vi "Front IO Panel.vi"(11 "Full System Configuration":T1={"Rack"=enum."15U; 1-Phase; 16A; 100-240V", "Middle Rail"=enum."None", "Ballast"={"Main"=0, "Small"=0, "Side"=0}, "Front Panel I/O"={"EMO Button"=FALSE, "USB 3.0"=FALSE, "Display"=FALSE, "1st USB 2.0"=FALSE, "2nd USB 2.0"=FALSE, "Ethernet 3"=FALSE, "EMO Extension (3rd Party)"=FALSE, "EMO Extension (Rack In & Out)"=FALSE, "Aux Dual C13 QAC Outlets"=FALSE, "Residual-current Circuit Breaker"=FALSE, "Serial"=FALSE, "GPIB"=FALSE}, "Rear Panel I/O"={"Rear Panel I/O Configuration"=enum."Blank Panel", "EMO Button"=FALSE, "Power, Status & Banana Ground"=FALSE, "Ethernet 2"=FALSE, "Display"=FALSE, "USB 3.0"=FALSE, "DIO"=FALSE, "GPIB"=FALSE, "Aux Dual C13 QAC Outlets"=FALSE, "Residual-current Circuit Breaker"=FALSE, "Serial"=FALSE, "SMA"=FALSE}, "Miscellaneous Options"={"Eyebolts"=FALSE, "Tower Light"=FALSE, "Top/Side Monitor Mount Kit"=FALSE, "24\" Monitor"=FALSE, "Keyboard & Mouse"=FALSE, "Secondary Ethernet Switch"=FALSE, "Extra USB Hub"=FALSE, "USB-6509"=FALSE, "Front Door"=enum."38U (Solid) IG", "Primary Ethernet Switch"=enum."Item 0", "Use Posture"=enum."Item 0"}, "Accessories"={"Screw Type"=enum."10-32", "Cage Nuts & Screws"=0.0, "Filler Panel Color"=enum."Interface Gray", "1U"=0.0, "2U"=0.0, "3U"=0.0}} {"Ballast"."Side" max=5 step=1; "Ballast"."Small" max=5 step=1; "Ballast"."Main" max=5 step=1}) -> (3 "Array":T13[](array[typedef]))   [LabVIEW 2023]
uses:
  Option Type Defs/Parts List.ctl
  Option Type Defs/Full System Configuration.ctl
  Option Type Defs/Rack.ctl
  Option Type Defs/Middle Rail.ctl
  Option Type Defs/Ballast.ctl
  Option Type Defs/Front Panel IO.ctl
  Option Type Defs/Rear Panel IO.ctl
  Option Type Defs/Rear Panel IO Configuration.ctl
  Option Type Defs/Miscellaneous Options.ctl
  Option Type Defs/Front Door.ctl
  Option Type Defs/Accessories.ctl
  Option Type Defs/Screw Types.ctl
  Option Type Defs/Filler Panel Color.ctl
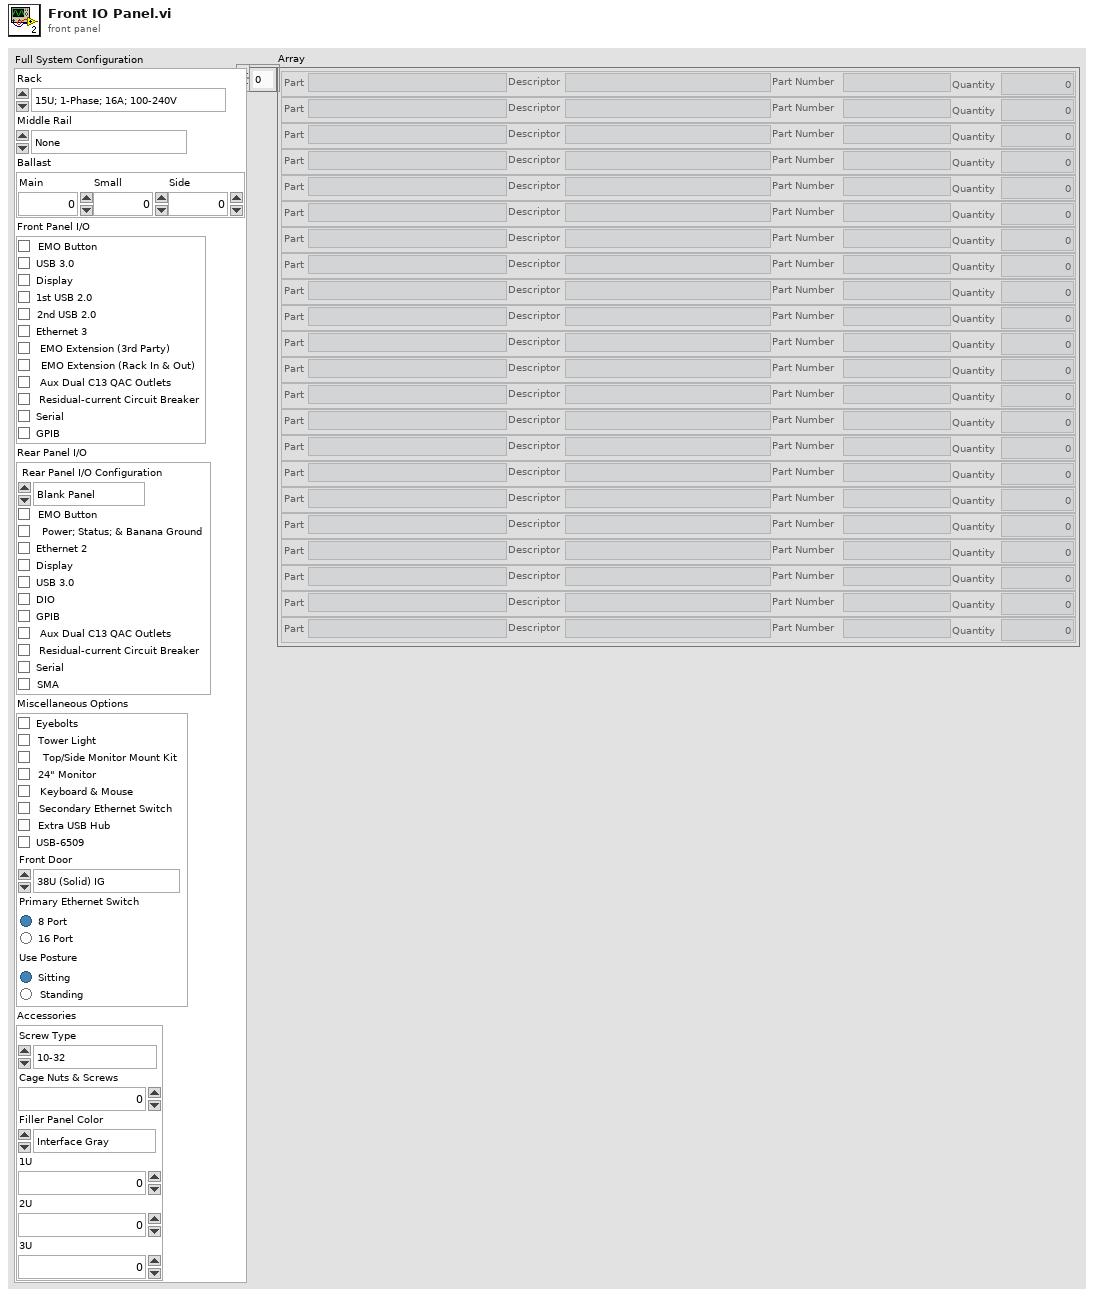
[diagram p1: front panel]
types:
  T1 = typedef "Full System Configuration.ctl" = cluster{"Rack":T2, "Middle Rail":T3, "Ballast":T4, "Front Panel I/O":T5, "Rear Panel I/O":T6, "Miscellaneous Options":T8, "Accessories":T10}
  T2 = typedef "Rack.ctl" = enum16{"15U; 1-Phase; 16A; 100-240V", "15U; 1-Phase; 24A; 100-240V", "38U; 3-Phase Delta; 50A; 200-240V", "38U; 1-Phase; 24A; 100-120V", "38U; 3-Phase Wye; 50A; 200-240V", "38U; 3-Phase Delta; 50A; 380-480V", "38U; 3-Phase Delta; 32A; 200-240V", "38U; 3-Phase Wye; 16A; 100-240V", "44U; 1-Phase; 24A; 100-240V", "44U; 3-Phase Delta; 32A; 200-240V"}
  T3 = typedef "Middle Rail.ctl" = enum16{"None", "Flip Side Rear; D=168.83mm", "Parallel Rear; D=145mm", "Flip Side Front; D=145mm", "Parallel Front; D=145mm"}
  T4 = typedef "Ballast.ctl" = cluster{"Main":u16, "Small":u16, "Side":u16}
  T5 = typedef "Front Panel IO.ctl" = cluster{"EMO Button":bool, "USB 3.0":bool, "Display":bool, "1st USB 2.0":bool, "2nd USB 2.0":bool, "Ethernet 3":bool, "EMO Extension (3rd Party)":bool, "EMO Extension (Rack In & Out)":bool, "Aux Dual C13 QAC Outlets":bool, "Residual-current Circuit Breaker":bool, "Serial":bool, "GPIB":bool}
  T6 = typedef "Rear Panel IO.ctl" = cluster{"Rear Panel I/O Configuration":T7, "EMO Button":bool, "Power, Status & Banana Ground":bool, "Ethernet 2":bool, "Display":bool, "USB 3.0":bool, "DIO":bool, "GPIB":bool, "Aux Dual C13 QAC Outlets":bool, "Residual-current Circuit Breaker":bool, "Serial":bool, "SMA":bool}
  T7 = typedef "Rear Panel IO Configuration.ctl" = enum16{"Blank Panel", "Fully Populated Panel", "Custom Panel"}
  T8 = typedef "Miscellaneous Options.ctl" = cluster{"Eyebolts":bool, "Tower Light":bool, "Top/Side Monitor Mount Kit":bool, "24\" Monitor":bool, "Keyboard & Mouse":bool, "Secondary Ethernet Switch":bool, "Extra USB Hub":bool, "USB-6509":bool, "Front Door":T9, "Primary Ethernet Switch":enum32{"Item 0", "Item 1"}, "Use Posture":enum32{"Item 0", "Item 1"}}
  T9 = typedef "Front Door.ctl" = enum16{"None", "38U (Solid) IG", "38U (Solid) EG", "38U: Top 14U (Solid) IG", "38U (Clear) IG", "44U (Solid) IG", "44U (Solid) EG"}
  T10 = typedef "Accessories.ctl" = cluster{"Screw Type":T11, "Cage Nuts & Screws":dbl, "Filler Panel Color":T12, "1U":dbl, "2U":dbl, "3U":dbl}
  T11 = typedef "Screw Types.ctl" = enum16{"None", "M6 (Most Common)", "10-32", "12-24"}
  T12 = typedef "Filler Panel Color.ctl" = enum16{"None", "Interface Gray", "Environmental Gray"}
  T13 = typedef "Parts List.ctl" = cluster{"Part":string, "Descriptor":string, "Part Number":string, "Quantity":dbl}
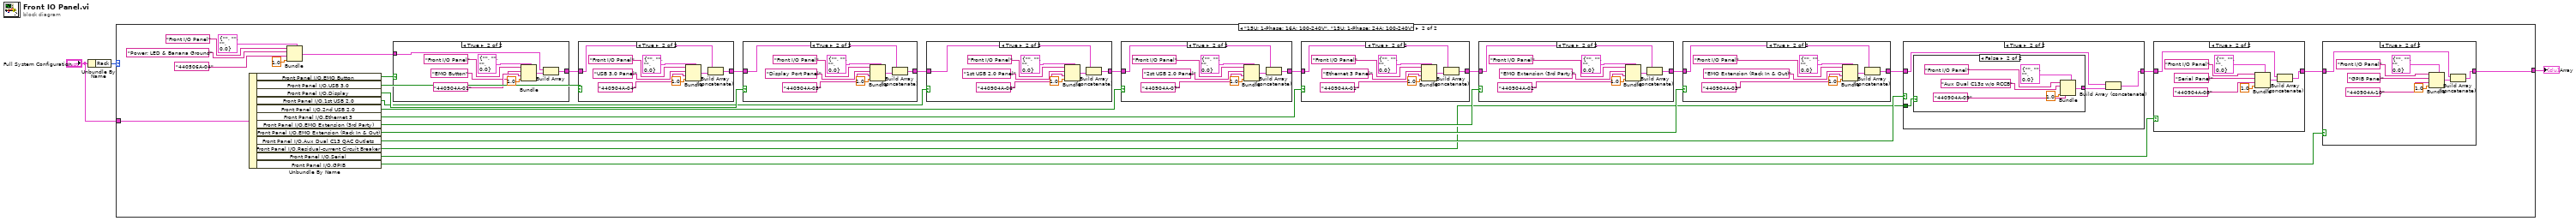
[diagram p0: block diagram]
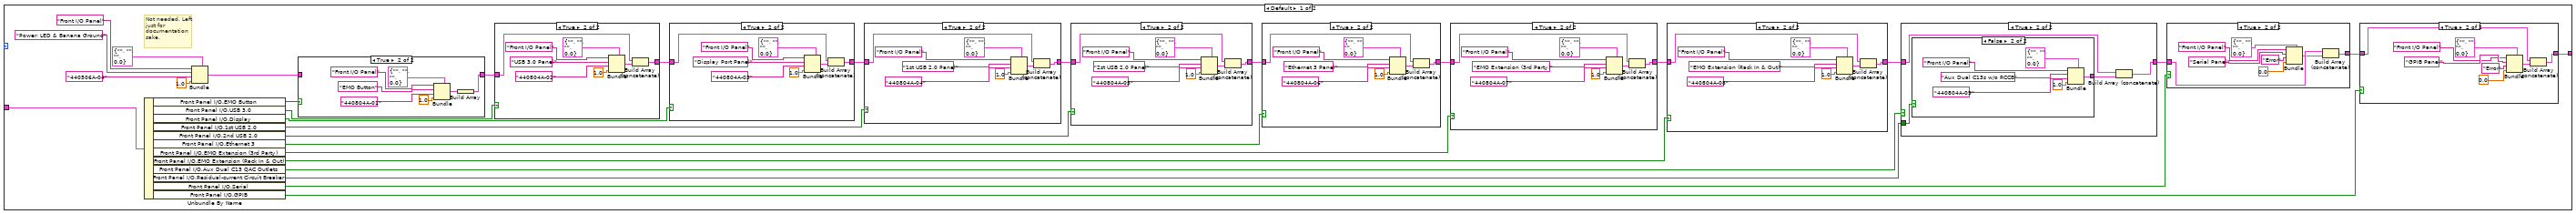
[diagram p2: hidden frame]
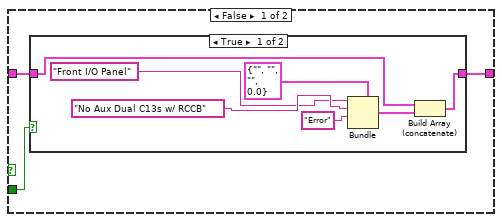
[diagram p5: hidden frame]
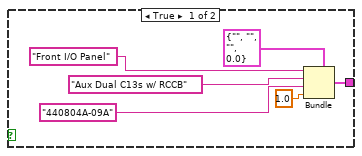
[diagram p7: hidden frame]
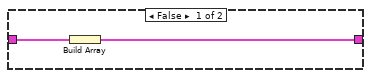
[diagram p15: hidden frame]
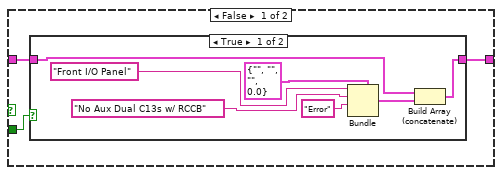
[diagram p18: hidden frame]
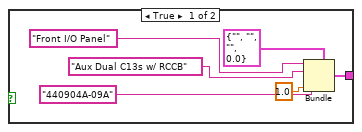
[diagram p20: hidden frame]
diagram:
  n1 = Unbundle By Name("Full System Configuration") -> ("Rack"=w3:T2)
  n2 = case shown="\"15U; 1-Phase; 16A; 100-240V\", \"15U; 1-Phase; 24A; 100-240V\"" w3 {
    tunnel: [w5 w152] -> w2
    tunnel: "Full System Configuration" -> [w28 w175]
    frame Default {
      # "Not needed. Left just for documentation sake."
      n3 = Unbundle By Name(w28) -> ("Front Panel I/O.EMO Button"=w27:bool, "Front Panel I/O.USB 3.0"=w26:bool, "Front Panel I/O.Display"=w23:bool, "Front Panel I/O.1st USB 2.0"=w21:bool, "Front Panel I/O.2nd USB 2.0"=w20:bool, "Front Panel I/O.Ethernet 3"=w18:bool, "Front Panel I/O.EMO Extension (3rd Party)"=w15:bool, "Front Panel I/O.EMO Extension (Rack In & Out)"=w13:bool, "Front Panel I/O.Aux Dual C13 QAC Outlets"=w12:bool, "Front Panel I/O.Residual-current Circuit Breaker"=w11:bool, "Front Panel I/O.Serial"=w7:bool, "Front Panel I/O.GPIB"=w6:bool)
      n4 = Bundle(cluster=T13 {"Part"="", "Descriptor"="", "Part Number"="", "Quantity"=0.0}, "Part"="Front I/O Panel", "Descriptor"="Power; LED & Banana Ground", "Part Number"="440506A-04", "Quantity"=1.0) -> (w33:T13)
      n5 = case shown="True" w27 {
        tunnel: w33 -> [w143 _]
        tunnel: [w142 w150] -> w25
        frame False {
          n6 = Build Array(w143) -> (w142:T13[])
        }
        frame True {
          n7 = Bundle(cluster=T13 {"Part"="", "Descriptor"="", "Part Number"="", "Quantity"=0.0}, "Part"="Front I/O Panel", "Descriptor"="EMO Button", "Part Number"="440804A-01", "Quantity"=1.0) -> (w145:T13)
          n8 = Build Array(w145) -> (w150:T13[])
        }
      }
      n9 = case shown="True" w26 {
        tunnel: w25 -> [w133 w141]
        tunnel: [w133 w140] -> w24
        frame False {
        }
        frame True {
          n10 = Bundle(cluster=T13 {"Part"="", "Descriptor"="", "Part Number"="", "Quantity"=0.0}, "Part"="Front I/O Panel", "Descriptor"="USB 3.0 Panel", "Part Number"="440804A-02", "Quantity"=1.0) -> (w135:T13)
          n11 = Build Array (concatenate)(w141, w135) -> (w140:T13[])
        }
      }
      n12 = case shown="True" w23 {
        tunnel: w24 -> [w124 w132]
        tunnel: [w124 w131] -> w22
        frame False {
        }
        frame True {
          n13 = Bundle(cluster=T13 {"Part"="", "Descriptor"="", "Part Number"="", "Quantity"=0.0}, "Part"="Front I/O Panel", "Descriptor"="Display Port Panel", "Part Number"="440804A-03", "Quantity"=1.0) -> (w126:T13)
          n14 = Build Array (concatenate)(w132, w126) -> (w131:T13[])
        }
      }
      n15 = case shown="True" w21 {
        tunnel: w22 -> [w115 w123]
        tunnel: [w115 w122] -> w19
        frame False {
        }
        frame True {
          n16 = Bundle(cluster=T13 {"Part"="", "Descriptor"="", "Part Number"="", "Quantity"=0.0}, "Part"="Front I/O Panel", "Descriptor"="1st USB 2.0 Panel", "Part Number"="440804A-04", "Quantity"=1.0) -> (w117:T13)
          n17 = Build Array (concatenate)(w123, w117) -> (w122:T13[])
        }
      }
      n18 = case shown="True" w20 {
        tunnel: w19 -> [w106 w114]
        tunnel: [w106 w113] -> w17
        frame False {
        }
        frame True {
          n19 = Bundle(cluster=T13 {"Part"="", "Descriptor"="", "Part Number"="", "Quantity"=0.0}, "Part"="Front I/O Panel", "Descriptor"="2st USB 2.0 Panel", "Part Number"="440804A-05", "Quantity"=1.0) -> (w108:T13)
          n20 = Build Array (concatenate)(w114, w108) -> (w113:T13[])
        }
      }
      n21 = case shown="True" w18 {
        tunnel: w17 -> [w97 w105]
        tunnel: [w97 w104] -> w16
        frame False {
        }
        frame True {
          n22 = Bundle(cluster=T13 {"Part"="", "Descriptor"="", "Part Number"="", "Quantity"=0.0}, "Part"="Front I/O Panel", "Descriptor"="Ethernet 3 Panel", "Part Number"="440804A-06", "Quantity"=1.0) -> (w99:T13)
          n23 = Build Array (concatenate)(w105, w99) -> (w104:T13[])
        }
      }
      n24 = case shown="True" w15 {
        tunnel: w16 -> [w88 w96]
        tunnel: [w88 w95] -> w14
        frame False {
        }
        frame True {
          n25 = Bundle(cluster=T13 {"Part"="", "Descriptor"="", "Part Number"="", "Quantity"=0.0}, "Part"="Front I/O Panel", "Descriptor"="EMO Extension (3rd Party)", "Part Number"="440804A-07", "Quantity"=1.0) -> (w90:T13)
          n26 = Build Array (concatenate)(w96, w90) -> (w95:T13[])
        }
      }
      n27 = case shown="True" w13 {
        tunnel: w14 -> [w79 w87]
        tunnel: [w79 w86] -> w10
        frame False {
        }
        frame True {
          n28 = Bundle(cluster=T13 {"Part"="", "Descriptor"="", "Part Number"="", "Quantity"=0.0}, "Part"="Front I/O Panel", "Descriptor"="EMO Extension (Rack In & Out)", "Part Number"="440804A-08", "Quantity"=1.0) -> (w81:T13)
          n29 = Build Array (concatenate)(w87, w81) -> (w86:T13[])
        }
      }
      n30 = case shown="True" w12 {
        tunnel: w10 -> [w53 w66]
        tunnel: [w52 w65] -> w8
        tunnel: w11 -> [w54 w63]
        frame False {
          n31 = case shown="True" w54 {
            tunnel: w53 -> [w57 w62]
            tunnel: [w56 w62] -> w52
            frame True {
              n32 = Bundle(cluster=T13 {"Part"="", "Descriptor"="", "Part Number"="", "Quantity"=0.0}, "Part"="Front I/O Panel", "Descriptor"="No Aux Dual C13s w/ RCCB", "Part Number"="Error") -> (w55:T13)  [unwired: 1 in]
              n33 = Build Array (concatenate)(w57, w55) -> (w56:T13[])
            }
            frame False {
            }
          }
        }
        frame True {
          n34 = case shown="False" w63 {
            tunnel: [w68 w74] -> w64
            frame True {
              n35 = Bundle(cluster=T13 {"Part"="", "Descriptor"="", "Part Number"="", "Quantity"=0.0}, "Part"="Front I/O Panel", "Descriptor"="Aux Dual C13s w/ RCCB", "Part Number"="440804A-09A", "Quantity"=1.0) -> (w68:T13)
            }
            frame False {
              n36 = Bundle(cluster=T13 {"Part"="", "Descriptor"="", "Part Number"="", "Quantity"=0.0}, "Part"="Front I/O Panel", "Descriptor"="Aux Dual C13s w/o RCCB", "Part Number"="440804A-09", "Quantity"=1.0) -> (w74:T13)
            }
          }
          n37 = Build Array (concatenate)(w66, w64) -> (w65:T13[])
        }
      }
      n38 = case shown="True" w7 {
        tunnel: w8 -> [w43 w51]
        tunnel: [w43 w50] -> w9
        frame False {
        }
        frame True {
          n39 = Bundle(cluster=T13 {"Part"="", "Descriptor"="", "Part Number"="", "Quantity"=0.0}, "Part"="Front I/O Panel", "Descriptor"="Serial Panel", "Part Number"="Error", "Quantity"=0.0) -> (w45:T13)
          n40 = Build Array (concatenate)(w51, w45) -> (w50:T13[])
        }
      }
      n41 = case shown="True" w6 {
        tunnel: w9 -> [w34 w42]
        tunnel: [w34 w41] -> w5
        frame False {
        }
        frame True {
          n42 = Bundle(cluster=T13 {"Part"="", "Descriptor"="", "Part Number"="", "Quantity"=0.0}, "Part"="Front I/O Panel", "Descriptor"="GPIB Panel", "Part Number"="Error", "Quantity"=0.0) -> (w36:T13)
          n43 = Build Array (concatenate)(w42, w36) -> (w41:T13[])
        }
      }
    }
    frame "15U; 1-Phase; 16A; 100-240V", "15U; 1-Phase; 24A; 100-240V" {
      n44 = Unbundle By Name(w175) -> ("Front Panel I/O.EMO Button"=w174:bool, "Front Panel I/O.USB 3.0"=w173:bool, "Front Panel I/O.Display"=w170:bool, "Front Panel I/O.1st USB 2.0"=w168:bool, "Front Panel I/O.2nd USB 2.0"=w167:bool, "Front Panel I/O.Ethernet 3"=w165:bool, "Front Panel I/O.EMO Extension (3rd Party)"=w162:bool, "Front Panel I/O.EMO Extension (Rack In & Out)"=w160:bool, "Front Panel I/O.Aux Dual C13 QAC Outlets"=w159:bool, "Front Panel I/O.Residual-current Circuit Breaker"=w158:bool, "Front Panel I/O.Serial"=w156:bool, "Front Panel I/O.GPIB"=w155:bool)
      n45 = Bundle(cluster=T13 {"Part"="", "Descriptor"="", "Part Number"="", "Quantity"=0.0}, "Part"="Front I/O Panel", "Descriptor"="Power; LED & Banana Ground", "Part Number"="440506A-04", "Quantity"=1.0) -> (w180:T13)
      n46 = case shown="True" w174 {
        tunnel: w180 -> [w290 w298]
        tunnel: [w289 w297] -> w172
        frame False {
          n47 = Build Array(w290) -> (w289:T13[])
        }
        frame True {
          n48 = Bundle(cluster=T13 {"Part"="", "Descriptor"="", "Part Number"="", "Quantity"=0.0}, "Part"="Front I/O Panel", "Descriptor"="EMO Button", "Part Number"="440904A-01", "Quantity"=1.0) -> (w292:T13)
          n49 = Build Array(w298, w292) -> (w297:T13[])
        }
      }
      n50 = case shown="True" w173 {
        tunnel: w172 -> [w280 w288]
        tunnel: [w280 w287] -> w171
        frame False {
        }
        frame True {
          n51 = Bundle(cluster=T13 {"Part"="", "Descriptor"="", "Part Number"="", "Quantity"=0.0}, "Part"="Front I/O Panel", "Descriptor"="USB 3.0 Panel", "Part Number"="440904A-04", "Quantity"=1.0) -> (w282:T13)
          n52 = Build Array (concatenate)(w288, w282) -> (w287:T13[])
        }
      }
      n53 = case shown="True" w170 {
        tunnel: w171 -> [w271 w279]
        tunnel: [w271 w278] -> w169
        frame False {
        }
        frame True {
          n54 = Bundle(cluster=T13 {"Part"="", "Descriptor"="", "Part Number"="", "Quantity"=0.0}, "Part"="Front I/O Panel", "Descriptor"="Display Port Panel", "Part Number"="440904A-05", "Quantity"=1.0) -> (w273:T13)
          n55 = Build Array (concatenate)(w279, w273) -> (w278:T13[])
        }
      }
      n56 = case shown="True" w168 {
        tunnel: w169 -> [w262 w270]
        tunnel: [w262 w269] -> w166
        frame False {
        }
        frame True {
          n57 = Bundle(cluster=T13 {"Part"="", "Descriptor"="", "Part Number"="", "Quantity"=0.0}, "Part"="Front I/O Panel", "Descriptor"="1st USB 2.0 Panel", "Part Number"="440904A-06", "Quantity"=1.0) -> (w264:T13)
          n58 = Build Array (concatenate)(w270, w264) -> (w269:T13[])
        }
      }
      n59 = case shown="True" w167 {
        tunnel: w166 -> [w253 w261]
        tunnel: [w253 w260] -> w164
        frame False {
        }
        frame True {
          n60 = Bundle(cluster=T13 {"Part"="", "Descriptor"="", "Part Number"="", "Quantity"=0.0}, "Part"="Front I/O Panel", "Descriptor"="2st USB 2.0 Panel", "Part Number"="440904A-07", "Quantity"=1.0) -> (w255:T13)
          n61 = Build Array (concatenate)(w261, w255) -> (w260:T13[])
        }
      }
      n62 = case shown="True" w165 {
        tunnel: w164 -> [w244 w252]
        tunnel: [w244 w251] -> w163
        frame False {
        }
        frame True {
          n63 = Bundle(cluster=T13 {"Part"="", "Descriptor"="", "Part Number"="", "Quantity"=0.0}, "Part"="Front I/O Panel", "Descriptor"="Ethernet 3 Panel", "Part Number"="440904A-01", "Quantity"=1.0) -> (w246:T13)
          n64 = Build Array (concatenate)(w252, w246) -> (w251:T13[])
        }
      }
      n65 = case shown="True" w162 {
        tunnel: w163 -> [w235 w243]
        tunnel: [w235 w242] -> w161
        frame False {
        }
        frame True {
          n66 = Bundle(cluster=T13 {"Part"="", "Descriptor"="", "Part Number"="", "Quantity"=0.0}, "Part"="Front I/O Panel", "Descriptor"="EMO Extension (3rd Party)", "Part Number"="440904A-02", "Quantity"=1.0) -> (w237:T13)
          n67 = Build Array (concatenate)(w243, w237) -> (w242:T13[])
        }
      }
      n68 = case shown="True" w160 {
        tunnel: w161 -> [w226 w234]
        tunnel: [w226 w233] -> w157
        frame False {
        }
        frame True {
          n69 = Bundle(cluster=T13 {"Part"="", "Descriptor"="", "Part Number"="", "Quantity"=0.0}, "Part"="Front I/O Panel", "Descriptor"="EMO Extension (Rack In & Out)", "Part Number"="440904A-03", "Quantity"=1.0) -> (w228:T13)
          n70 = Build Array (concatenate)(w234, w228) -> (w233:T13[])
        }
      }
      n71 = case shown="True" w159 {
        tunnel: w157 -> [w200 w213]
        tunnel: [w199 w212] -> w154
        tunnel: w158 -> [w201 w210]
        frame False {
          n72 = case shown="True" w201 {
            tunnel: w200 -> [w204 w209]
            tunnel: [w203 w209] -> w199
            frame True {
              n73 = Bundle(cluster=T13 {"Part"="", "Descriptor"="", "Part Number"="", "Quantity"=0.0}, "Part"="Front I/O Panel", "Descriptor"="No Aux Dual C13s w/ RCCB", "Part Number"="Error") -> (w202:T13)  [unwired: 1 in]
              n74 = Build Array (concatenate)(w204, w202) -> (w203:T13[])
            }
            frame False {
            }
          }
        }
        frame True {
          n75 = case shown="False" w210 {
            tunnel: [w215 w221] -> w211
            frame True {
              n76 = Bundle(cluster=T13 {"Part"="", "Descriptor"="", "Part Number"="", "Quantity"=0.0}, "Part"="Front I/O Panel", "Descriptor"="Aux Dual C13s w/ RCCB", "Part Number"="440904A-09A", "Quantity"=1.0) -> (w215:T13)
            }
            frame False {
              n77 = Bundle(cluster=T13 {"Part"="", "Descriptor"="", "Part Number"="", "Quantity"=0.0}, "Part"="Front I/O Panel", "Descriptor"="Aux Dual C13s w/o RCCB", "Part Number"="440904A-09", "Quantity"=1.0) -> (w221:T13)
            }
          }
          n78 = Build Array (concatenate)(w213, w211) -> (w212:T13[])
        }
      }
      n79 = case shown="True" w156 {
        tunnel: w154 -> [w190 w198]
        tunnel: [w190 w197] -> w153
        frame False {
        }
        frame True {
          n80 = Bundle(cluster=T13 {"Part"="", "Descriptor"="", "Part Number"="", "Quantity"=0.0}, "Part"="Front I/O Panel", "Descriptor"="Serial Panel", "Part Number"="440904A-08", "Quantity"=1.0) -> (w192:T13)
          n81 = Build Array (concatenate)(w198, w192) -> (w197:T13[])
        }
      }
      n82 = case shown="True" w155 {
        tunnel: w153 -> [w181 w189]
        tunnel: [w181 w188] -> w152
        frame False {
        }
        frame True {
          n83 = Bundle(cluster=T13 {"Part"="", "Descriptor"="", "Part Number"="", "Quantity"=0.0}, "Part"="Front I/O Panel", "Descriptor"="GPIB Panel", "Part Number"="440904A-10", "Quantity"=1.0) -> (w183:T13)
          n84 = Build Array (concatenate)(w189, w183) -> (w188:T13[])
        }
      }
    }
  }
  "Array" <- w2
